vi "autonstand.vi"() -> ()   [LabVIEW 2012, in "Robohawks White.lvrbt"]
uses:
  Robohawks White.lvrbt
  <vilib>/NXT/Hardware/Plugins/Tetrix DC Motor/TetrixDCMotorAddress.ctl
  <vilib>/NXT/Block Support/NXT_InputPort.ctl
  <vilib>/NXT/HiTechnic/HiTechnic Controls/HiTechnic Port.ctl
  <vilib>/NXT/NXTIO Xnodes/NXTIONodeSubVIs/TETRIX IO Check Battery.vi
  <vilib>/NXT/Dual Mode Library/Waits/Wait_Num(msec).vi
  <vilib>/NXT/NXTIO Xnodes/NXTIONodeSubVIs/TETRIX IO Stop DC Motors.vi
  <vilib>/NXT/Dual Mode Library/Waits/Wait_Num.vi
  <vilib>/NXT/NXTIO Xnodes/NXTIONodeSubVIs/TETRIX IO Move DC Motors.vi
  <vilib>/NXT/HiTechnic/HiTechnic Read/HiTechnic IRSeeker Sensor_V1 all.vi
  <vilib>/NXT/Dual Mode Library/Sound/PlayRedPianoFile.vi
  <vilib>/NXT/Dual Mode Library/Sound/PlayGreenPianoFile.vi
  <vilib>/NXT/Dual Mode Library/Sound/PlayBluePianoFile.vi
  <vilib>/NXT/Subs/LVHSConnector.ctl
  <vilib>/NXT/NXTIO Xnodes/AddressXNode/NXTIOAddress.xnode
  <vilib>/NXT/NXTIO Xnodes/NXTIOXNode/NXTIO.xnode
  <vilib>/NXT/LegoClasses/BrickReference/BrickReference.lvclass
panel:
  out "Enabled":bool
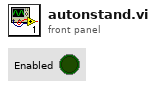
[diagram p1: front panel]
types:
  T1 = typedef "TetrixDCMotorAddress.ctl" = i32
  T2 = typedef "LVHSConnector.ctl" = refnum<class "BrickReference.lvclass">
  T3 = typedef "HiTechnic Port.ctl" = cluster{"Port":T4, "MUX Port":u8}
  T4 = typedef "NXT_InputPort.ctl" = u32
  T5 = cluster{"Direction (0-9)":i16, "Signal Strength (Array)":u8[]}
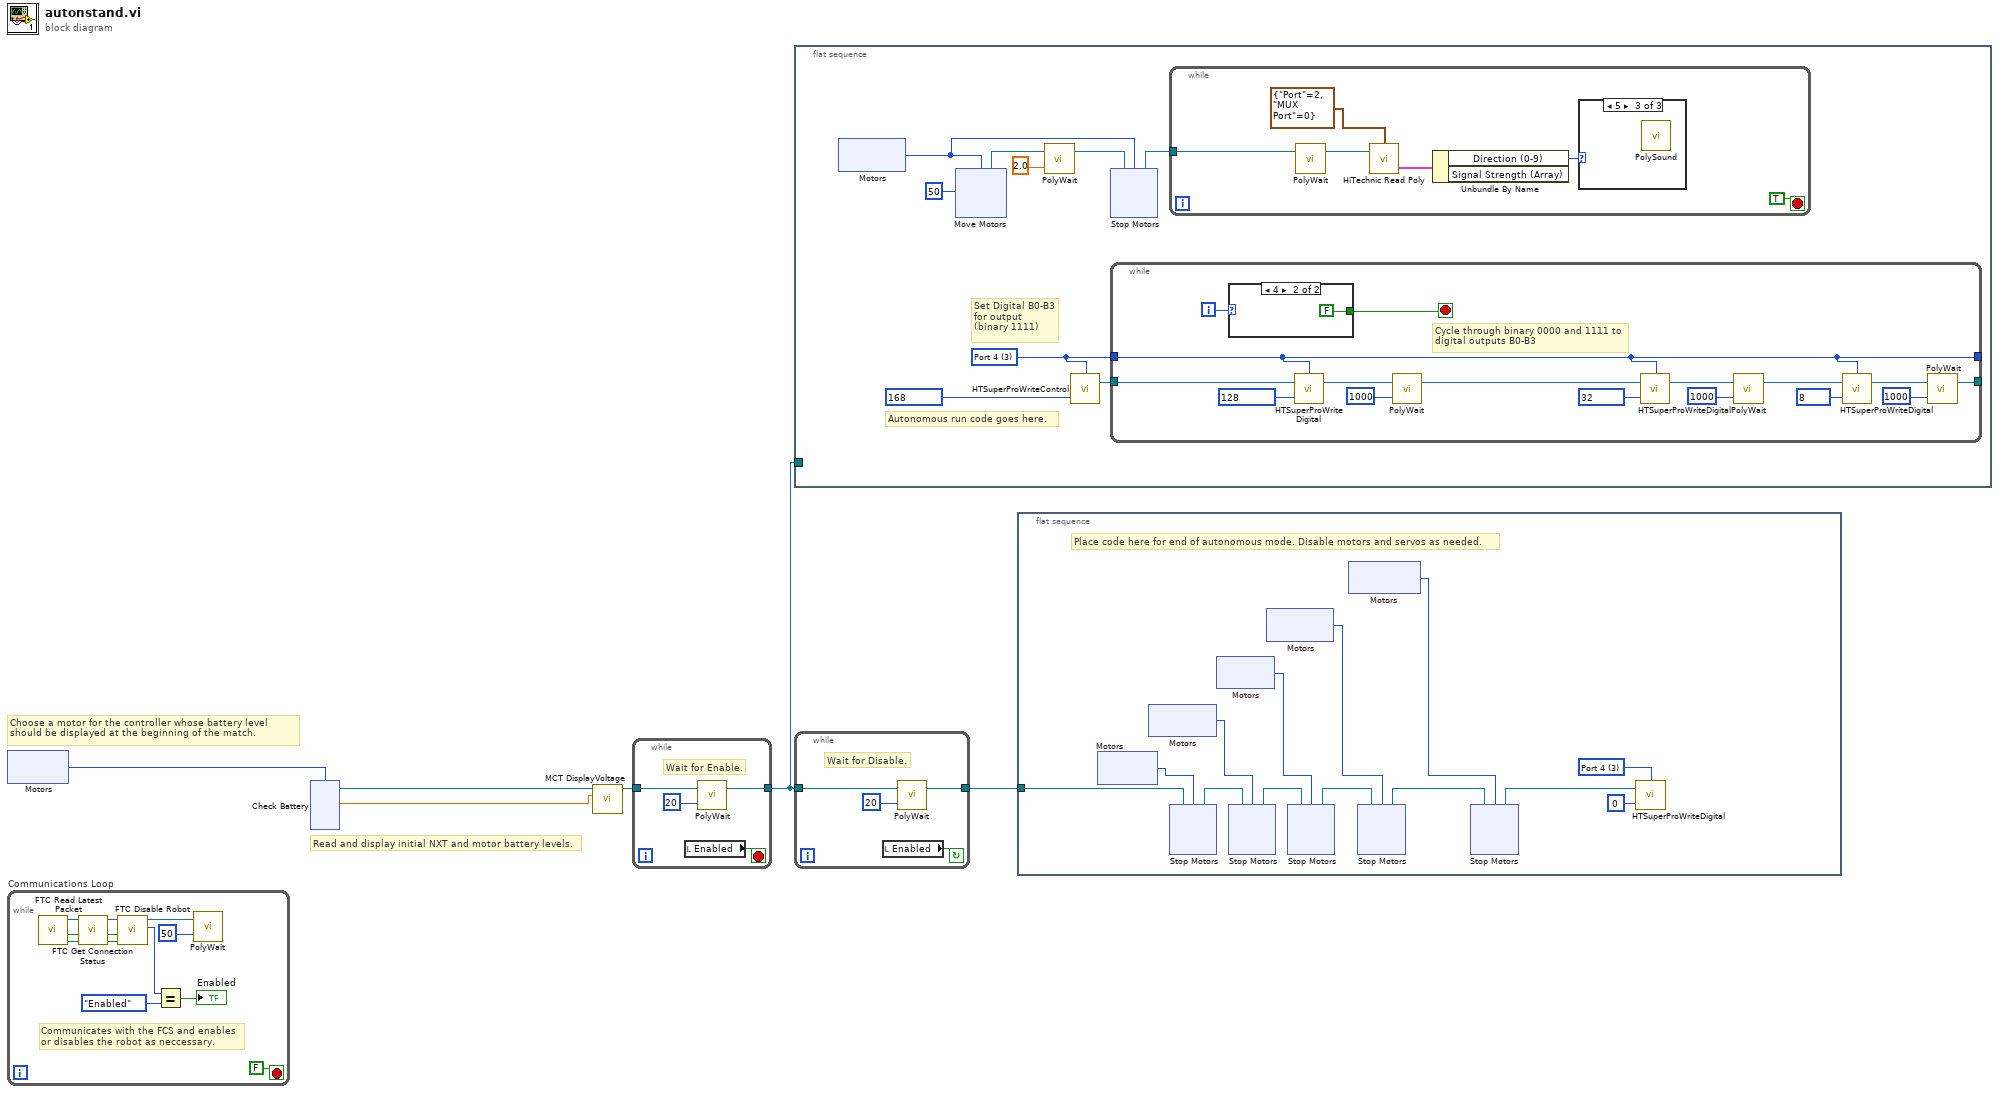
[diagram p0: block diagram]
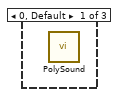
[diagram p2: hidden frame]
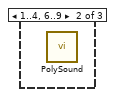
[diagram p3: hidden frame]
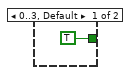
[diagram p4: hidden frame]
diagram:
  # "Read and display initial NXT and motor battery levels."
  # "Choose a motor for the controller whose battery level \nshould be displayed at the beginning of the match."
  n1 = xnode "Motors"() -> ("Motor"=w1:T1)
  n2 = while "Communications Loop" {
    stop <- FALSE stop-if-true
    # "Communicates with the FCS and enables \nor disables the robot as neccessary."
    n3 = call <vilib>:"FTC Read Latest Packet.vi"() -> ("Packet Received?"=w16:bool, "Stopped?"=w15:bool, "NXT/EV3"=w18:T2)  [unwired: 6 in, 3 out]
    n4 = call <vilib>:"FTC Get Connection Status.vi"("Packet Received?"=w16, "Stopped?"=w15, "NXT/EV3"=w18) -> ("Online?"=w7:bool, "Stopped?"=w8:bool, "NXT/EV3"=w17:T2)  [unwired: 5 in]
    n5 = call <vilib>:"FTC Disable Robot.vi"("Online?"=w7, "Stopped?"=w8, "NXT/EV3"=w17) -> ("Enabled?"=w11:enum16{"Disabled", "Enabled"}, "NXT/EV3"=w13:T2)  [unwired: 3 in]
    n6 = Equal?(x=w11, y=enum16{"Disabled", "Enabled"}."Enabled") -> (x = y?=→"Enabled":bool)
    n7 = call-poly <vilib>:"PolyWait.vi"("Time (100 msec)"=u32 50 ("Time (msec)"), "NXT/EV3"=w13) -> ()  [unwired: 2 in, 1 out]
  }
  n8 = xnode "Check Battery"("Motors"=w1) -> ("Voltage 1"=w2:sgl, "NXT/EV3"=w4:T2)  [unwired: 1 in]
  n9 = call <vilib>:"MCT DisplayVoltage.vi"("Motor Voltage"=w2, "NXT/EV3"=w4) -> ("NXT/EV3"=w3:T2)  [unwired: 9 in]
  n10 = while {
    tunnel: [w20] -> w6
    tunnel: w3 -> [w19]
    stop <- w21 stop-if-true
    # "Wait for Enable."
    n11 = local read "Enabled"() -> (w21:bool)
    n12 = call-poly <vilib>:"PolyWait.vi"("Time (100 msec)"=u32 20 ("Time (msec)"), "NXT/EV3"=w19) -> ("NXT/EV3"=w20:T2)  [unwired: 2 in]
  }
  n13 = flat-sequence {
    tunnel: w6 -> [_]
    frame #0 {
      w29 = T4 3 items=["Port 1", "Port 2", "Port 3", "Port 4"] ("Port")
      # "Set Digital B0-B3\nfor output\n(binary 1111)"
      # "Autonomous run code goes here."
      n14 = xnode "Motors"() -> ("Motor"=w26:T1)
      n15 = xnode "Move Motors"("Power/Speed 1"=i8 50, "Motors"=w26) -> ("NXT/EV3"=w24:T2)  [unwired: 1 in]
      n16 = call-poly <vilib>:"PolyWait.vi"("Time (1 sec)"=sgl 2.0, "NXT/EV3"=w24) -> ("NXT/EV3"=w25:T2)  [unwired: 2 in]
      n17 = call "HTSuperProWriteControl.vi"("Digital Control"=u8 168, "Port"=w29) -> ("NXT"=w28:T2)  [unwired: 3 in]
      n18 = xnode "Stop Motors"("Motors"=w26, "NXT/EV3"=w25) -> ("NXT/EV3"=w23:T2)
      n19 = while {
        tunnel: w28 -> [w53]
        tunnel: w29 -> [w38]
        tunnel: [w39] -> _
        tunnel: [w38] -> _
        i -> [w40]
        stop <- w41 stop-if-true
        # "Cycle through binary 0000 and 1111 to\ndigital outputs B0-B3"
        n20 = case shown="4" w40 {
          tunnel: [TRUE FALSE] -> w41
          frame 0..3, Default {
          }
          frame 4 {
          }
        }
        n21 = call "HTSuperProWriteDigital.vi"("Digital Value"=u8 128 ("Digital Control"), "NXT"=w53, "Port"=w38) -> ("NXT"=w51:T2)  [unwired: 2 in]
        n22 = call-poly <vilib>:"PolyWait.vi"("Time (100 msec)"=u32 1000, "NXT/EV3"=w51) -> ("NXT/EV3"=w46:T2)  [unwired: 2 in]
        n23 = call "HTSuperProWriteDigital.vi"("Digital Value"=u8 32 ("Digital Control"), "NXT"=w46, "Port"=w38) -> ("NXT"=w48:T2)  [unwired: 2 in]
        n24 = call-poly <vilib>:"PolyWait.vi"("Time (100 msec)"=u32 1000, "NXT/EV3"=w48) -> ("NXT/EV3"=w42:T2)  [unwired: 2 in]
        n25 = call "HTSuperProWriteDigital.vi"("Digital Value"=u8 8 ("Digital Control"), "NXT"=w42, "Port"=w38) -> ("NXT"=w44:T2)  [unwired: 2 in]
        n26 = call-poly <vilib>:"PolyWait.vi"("Time (100 msec)"=u32 1000, "NXT/EV3"=w44) -> ("NXT/EV3"=w39:T2)  [unwired: 2 in]
      }
      n27 = while {
        tunnel: w23 -> [w36]
        stop <- TRUE stop-if-true
        n28 = call-poly <vilib>:"PolyWait.vi"("NXT/EV3"=w36) -> ("NXT/EV3"=w32:T2)  [unwired: 3 in]
        n29 = call-poly <vilib>:"HiTechnic Read Poly.vi"("NXT/EV3"=w32, "Port/MUX"=T3 {"Port"=2, "MUX Port"=0}) -> ("All Info"=w35:T5)  [unwired: 1 in, 1 out]
        n30 = Unbundle By Name(w35) -> ("Direction (0-9)"=w34:i16)  [unwired: 1 out]
        n31 = case shown="5" w34 {
          frame 0, Default {
            n32 = call-poly <vilib>:"PolySound.vi"() -> ()  [unwired: 4 in, 1 out]
          }
          frame 1..4, 6..9 {
            n33 = call-poly <vilib>:"PolySound.vi"() -> ()  [unwired: 4 in, 1 out]
          }
          frame 5 {
            n34 = call-poly <vilib>:"PolySound.vi"() -> ()  [unwired: 4 in, 1 out]
          }
        }
      }
    }
  }
  n35 = while {
    tunnel: [w70] -> w5
    tunnel: w6 -> [w69]
    stop <- w71 continue-if-true
    # "Wait for Disable."
    n36 = local read "Enabled"() -> (w71:bool)
    n37 = call-poly <vilib>:"PolyWait.vi"("Time (100 msec)"=u32 20 ("Time (msec)"), "NXT/EV3"=w69) -> ("NXT/EV3"=w70:T2)  [unwired: 2 in]
  }
  n38 = flat-sequence {
    tunnel: w5 -> [w73]
    frame #0 {
      w76 = T4 3 items=["Port 1", "Port 2", "Port 3", "Port 4"] ("Port")
      # "Place code here for end of autonomous mode. Disable motors and servos as needed."
      n39 = xnode "Motors"() -> ("Motor"=w85:T1)
      n40 = xnode "Motors"() -> ("Motor"=w84:T1)
      n41 = xnode "Stop Motors"("Motors"=w85, "NXT/EV3"=w73) -> ("NXT/EV3"=w82:T2)
      n42 = xnode "Motors"() -> ("Motor"=w83:T1)
      n43 = xnode "Stop Motors"("Motors"=w84, "NXT/EV3"=w82) -> ("NXT/EV3"=w81:T2)
      n44 = xnode "Motors"() -> ("Motor"=w80:T1)
      n45 = xnode "Stop Motors"("Motors"=w83, "NXT/EV3"=w81) -> ("NXT/EV3"=w79:T2)
      n46 = xnode "Motors"() -> ("Motor"=w78:T1)
      n47 = xnode "Stop Motors"("Motors"=w80, "NXT/EV3"=w79) -> ("NXT/EV3"=w77:T2)
      n48 = xnode "Stop Motors"("Motors"=w78, "NXT/EV3"=w77) -> ("NXT/EV3"=w75:T2)
      n49 = call "HTSuperProWriteDigital.vi"("Digital Value"=u8 0 ("Digital Control"), "NXT"=w75, "Port"=w76) -> ()  [unwired: 2 in, 1 out]
    }
  }
